vi "Controller FOFB Configuration In to Out.vi"(11 "LNLS Control FOFB Configuration In":T3={"Status"=0, "Operation Mode"=enum."Manual Mode", "Horizontal Gain"=0.0, "Vertical Gain"=0.0, "Selected Reference Orbit"=0, "Selected Correction Matrix"=0, "Selected FPGA Filters"=0, "Horizontal Distortion Threshold"=0.0, "Vertical Distortion Threshold"=0.0, "Fast Command Enabled"=FALSE, "Update Reference Orbit"=FALSE, "Update Contoller Configuration"=FALSE}) -> (3 "LNLS Control FOFB Configuration Out":T1={"Status"=0, "Operation Mode"=enum."Manual Mode", "Horizontal Gain"=0.0, "Vertical Gain"=0.0, "Selected Reference Orbit"=0, "Selected Correction Matrix"=0, "Selected FPGA Filters"=0, "Horizontal Distortion Threshold"=0.0, "Vertical Distortion Threshold"=0.0, "Timestamp"=0.0})   [LabVIEW 2011, in "Controller VIs.lvlib"]
uses:
  Controller VIs.lvlib
  Types Definitions/Type Control FOFB Configuration In.ctl
  Types Definitions/Type Operation Mode State.ctl
  Types Definitions/Type Control FOFB Configuration Out.ctl
  Type Definitions.lvlib
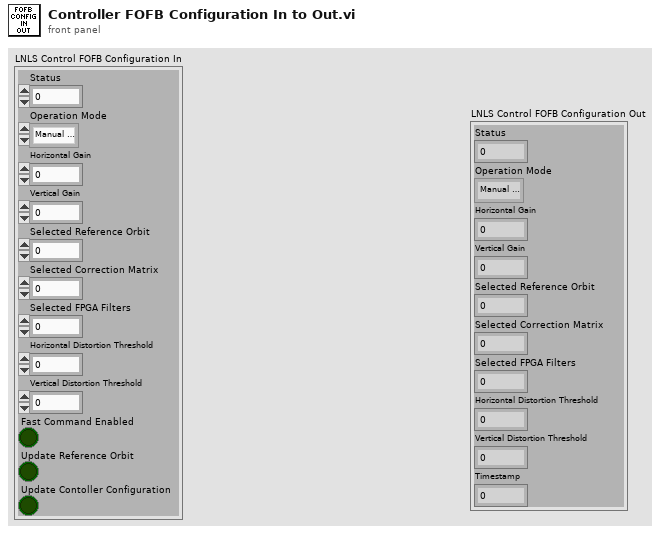
[diagram p1: front panel]
types:
  T1 = typedef "Type Definitions.lvlib/Type Control FOFB Configuration Out.ctl" = cluster{"Status":u16, "Operation Mode":T2, "Horizontal Gain":sgl, "Vertical Gain":sgl, "Selected Reference Orbit":i32, "Selected Correction Matrix":i32, "Selected FPGA Filters":i32, "Horizontal Distortion Threshold":sgl, "Vertical Distortion Threshold":sgl, "Timestamp":dbl}
  T2 = typedef "Type Definitions.lvlib/Type Operation Mode State.ctl" = enum8{"Idle Mode", "Manual Mode", "FOFB Mode"}
  T3 = typedef "Type Definitions.lvlib/Type Control FOFB Configuration In.ctl" = cluster{"Status":u16, "Operation Mode":T2, "Horizontal Gain":sgl, "Vertical Gain":sgl, "Selected Reference Orbit":i32, "Selected Correction Matrix":i32, "Selected FPGA Filters":i32, "Horizontal Distortion Threshold":sgl, "Vertical Distortion Threshold":sgl, "Fast Command Enabled":bool, "Update Reference Orbit":bool, "Update Contoller Configuration":bool}
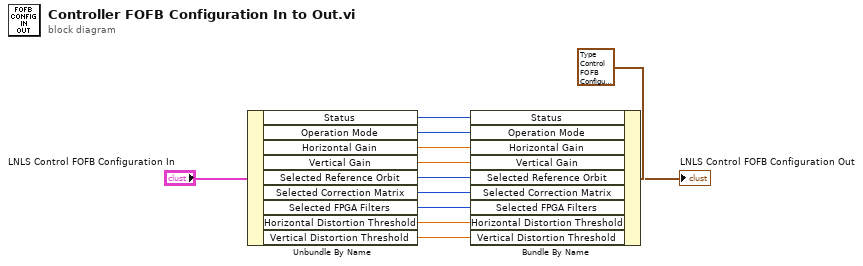
[diagram p0: block diagram]
diagram:
  n1 = Unbundle By Name("LNLS Control FOFB Configuration In") -> ("Status"=w12:u16, "Operation Mode"=w11:T2, "Horizontal Gain"=w10:sgl, "Vertical Gain"=w9:sgl, "Selected Reference Orbit"=w8:i32, "Selected Correction Matrix"=w7:i32, "Selected FPGA Filters"=w6:i32, "Horizontal Distortion Threshold"=w5:sgl, "Vertical Distortion Threshold"=w1:sgl)
  n2 = Bundle By Name(cluster=T1 {"Status"=0, "Operation Mode"=enum."Idle Mode", "Horizontal Gain"=0.0, "Vertical Gain"=0.0, "Selected Reference Orbit"=0, "Selected Correction Matrix"=0, "Selected FPGA Filters"=0, "Horizontal Distortion Threshold"=0.0, "Vertical Distortion Threshold"=0.0, "Timestamp"=0.0} ("LNLS Control FOFB Configuration Out"), "Status"=w12, "Operation Mode"=w11, "Horizontal Gain"=w10, "Vertical Gain"=w9, "Selected Reference Orbit"=w8, "Selected Correction Matrix"=w7, "Selected FPGA Filters"=w6, "Horizontal Distortion Threshold"=w5, "Vertical Distortion Threshold"=w1) -> (→"LNLS Control FOFB Configuration Out":T1)
